vi "arrayI32.vi"(2 "Array In":i32[](array[numeric]), 3 "Base":i32) -> (0 "Array Out (not in place)":i32[](array[numeric]), 1 "Array Out":i32[](array[numeric]))   [LabVIEW 2013]
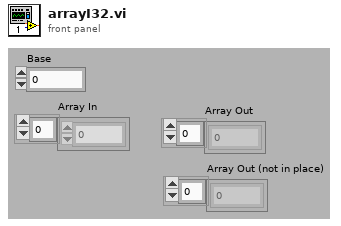
[diagram p1: front panel]
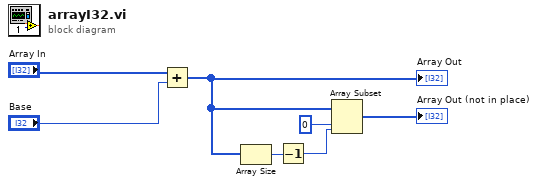
[diagram p0: block diagram]
diagram:
  n1 = Add(x="Array In", y="Base") -> (x+y=w2:i32[])
  "Array Out" <- w2
  n2 = Array Size(array=w2) -> (size(s)=w5:i32)
  n3 = Decrement(x=w5) -> (x-1=w6:i32)
  n4 = Array Subset(array=w2, index=0, length=w6) -> (→"Array Out (not in place)":i32[])
